vi "Kernel - Command Parser.vi"(7 "data in - Command Parser":T1, 8 "error in":errorcluster, 10 "state":string, 11 "message queue":refnum<queue>) -> (0 "error out":errorcluster, 3 "message queue (out)":refnum<queue>, 4 "stop?":bool, 5 "data out - Command Parser":T1)   [LabVIEW 2021]
uses:
  Typedefs/Data - Command Parser.ctl
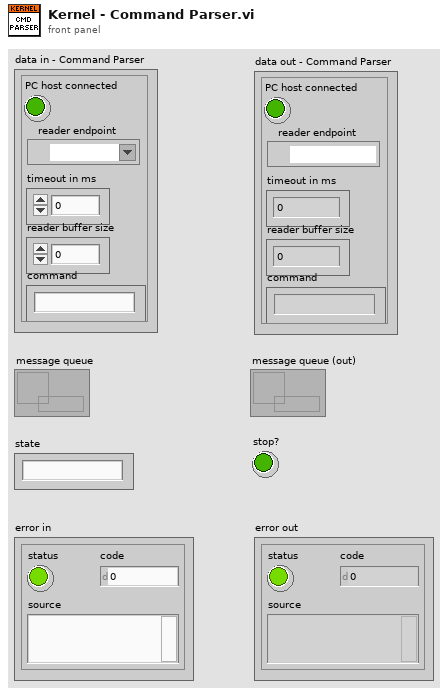
[diagram p1: front panel]
types:
  T1 = typedef "Data - Command Parser.ctl" = cluster{"PC host connected":bool, "timeout in ms":i32, "reader buffer size":i32, "command":string, "reader endpoint":refnum<k21>}
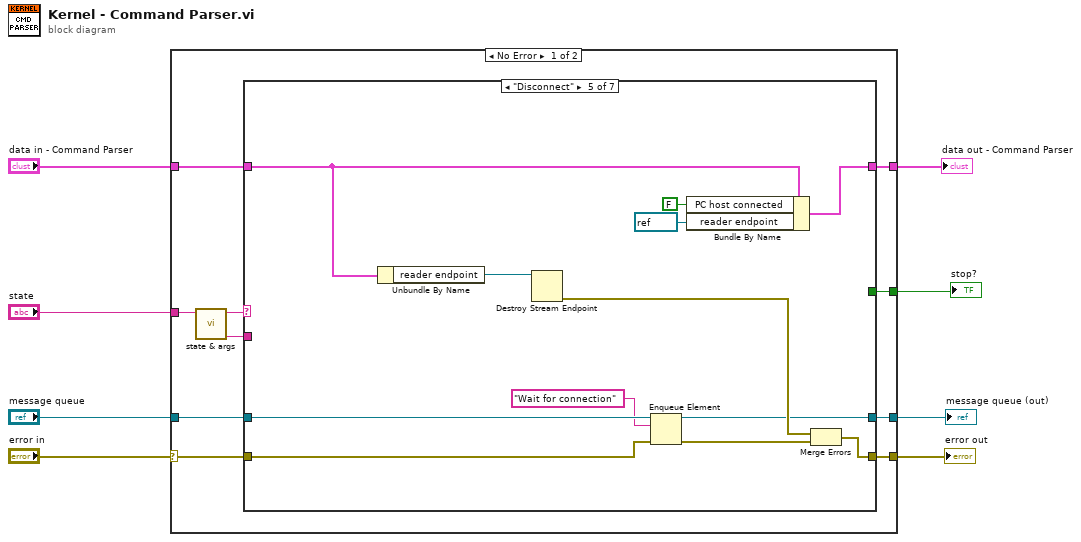
[diagram p0: block diagram]
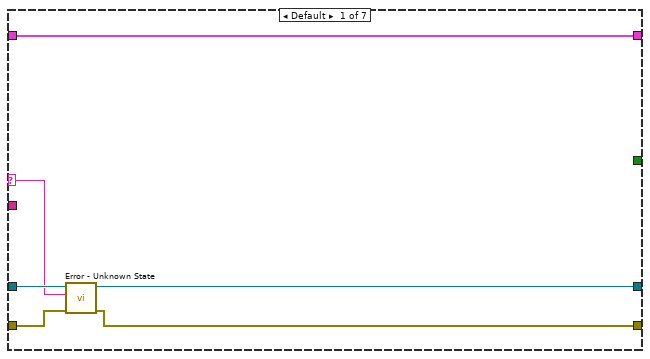
[diagram p2: hidden frame]
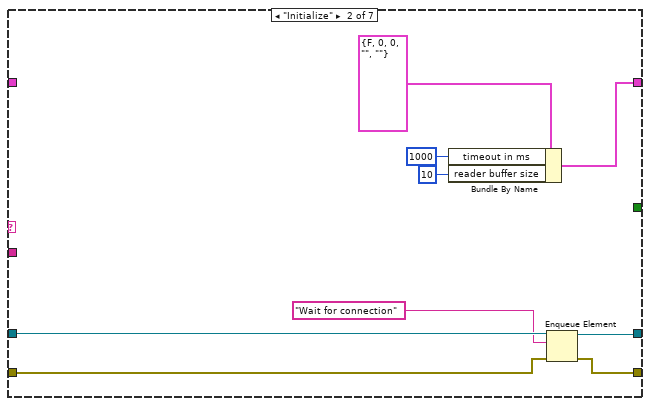
[diagram p3: hidden frame]
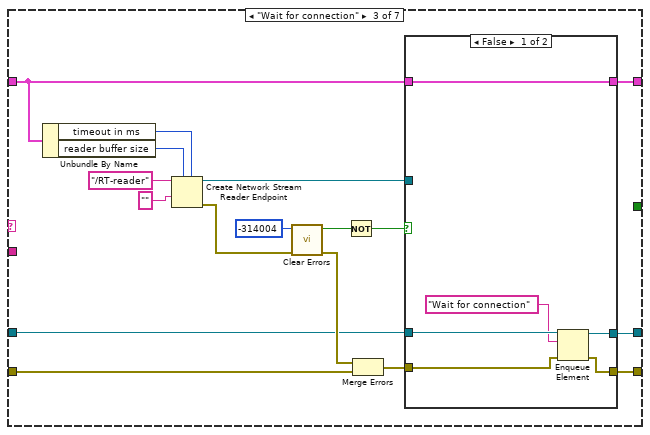
[diagram p4: hidden frame]
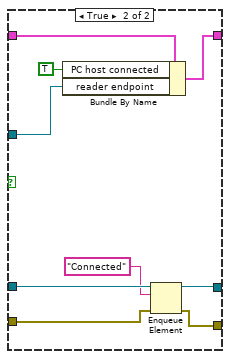
[diagram p5: hidden frame]
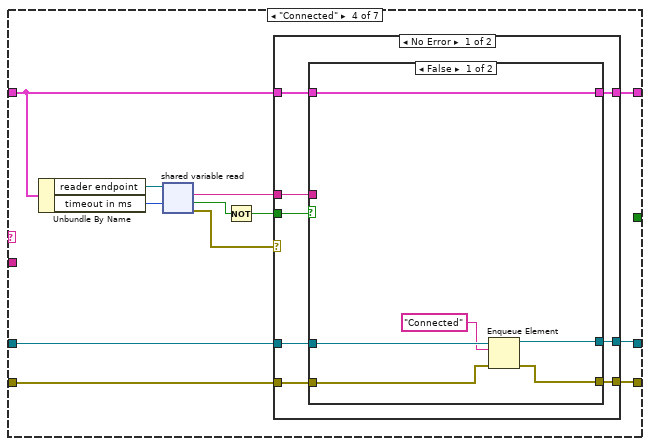
[diagram p6: hidden frame]
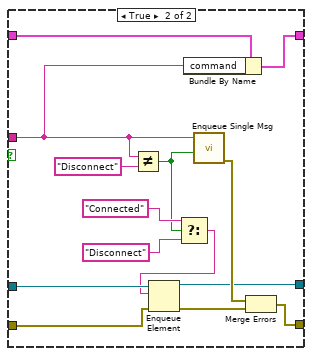
[diagram p7: hidden frame]
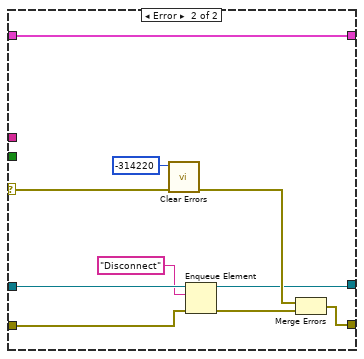
[diagram p8: hidden frame]
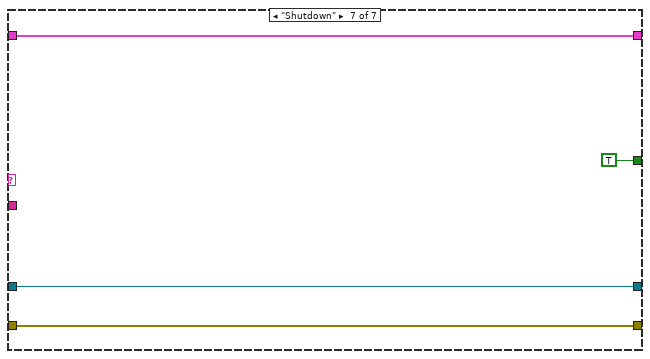
[diagram p10: hidden frame]
diagram:
  n1 = case shown="No Error" "error in" {
    selector: "error in" -> [w17 w135]
    tunnel: "message queue" -> [w18 w136]
    tunnel: "state" -> [w16 _]
    tunnel: "data in - Command Parser" -> [w13 w137]
    tunnel: [w12 w135] -> w4
    tunnel: [w11 w136] -> w3
    tunnel: [w10 w137] -> w2
    tunnel: [w9 _] -> w1
    frame No Error {
      n2 = call "state & args.vi"("state:args"=w16) -> ("args"=w14:string, "state"=w15:string)  [unwired: 9 in]
      n3 = case shown="\"Disconnect\"" w15 {
        selector: w15 -> [w21 _ _ _ _ _ _]
        tunnel: w18 -> [w23 w28 w34 w70 w121 w129 w133]
        tunnel: w17 -> [w24 w27 w39 w69 w117 w128 w134]
        tunnel: w14 -> [_ _ _ _ _ _ _]
        tunnel: w13 -> [w19 _ w49 w77 w124 w130 w132]
        tunnel: [w22 w29 w37 w68 w120 w129 w133] -> w11
        tunnel: [w20 w26 w36 w67 w118 w128 w134] -> w12
        tunnel: [w19 w30 w50 w66 w127 w130 w132] -> w10
        tunnel: [_ _ _ _ _ _ TRUE] -> w9
        frame Default {
          n4 = call "Error - Unknown State.vi"("error in"=w24, "state"=w21, "queue"=w23) -> ("error out"=w20:errorcluster, "queue out"=w22:refnum<queue>)  [unwired: 7 in]
        }
        frame "Initialize" {
          n5 = Bundle By Name(cluster=T1 {"PC host connected"=FALSE, "timeout in ms"=0, "reader buffer size"=0, "command"="", "reader endpoint"=""} ("data in - Command Parser"), "timeout in ms"=1000, "reader buffer size"=10) -> (w30:T1)
          n6 = Enqueue Element(queue=w28, element="Wait for connection", error in (no error)=w27) -> (queue out=w29:refnum<queue>, error out=w26:errorcluster)  [unwired: 1 in, 1 out]
        }
        frame "Wait for connection" {
          n7 = Unbundle By Name(w49) -> ("timeout in ms"=w48:i32, "reader buffer size"=w47:i32)
          n8 = Create Network Stream Reader Endpoint(5:w48, 7:w47, 9:"" ("writer url"), 11:"/RT-reader" ("reader name")) -> (0:w43:errorcluster, 3:w44:refnum<k21>)  [unwired: 3 in]
          n9 = call <vilib>:"Clear Errors.vi"("error in (no error)"=w43, "specific error code to clear (0: all)"=-314004) -> ("error out"=w38:errorcluster, "specific error cleared?"=w41:bool)  [unwired: 4 in]
          n10 = Not(x=w41) -> (.not. x?=w40:bool)
          n11 = Merge Errors(w38, w39) -> (w35:errorcluster)
          n12 = case shown="False" w40 {
            tunnel: w49 -> [w56 w65]
            tunnel: [w56 w64] -> w50
            tunnel: w44 -> [_ w62]
            tunnel: [w55 w61] -> w37
            tunnel: [w54 w58] -> w36
            tunnel: w35 -> [w53 w59]
            tunnel: w34 -> [w52 w60]
            frame False {
              n13 = Enqueue Element(queue=w52, element="Wait for connection", error in (no error)=w53) -> (queue out=w55:refnum<queue>, error out=w54:errorcluster)  [unwired: 1 in, 1 out]
            }
            frame True {
              n14 = Bundle By Name(cluster=w65, "PC host connected"=TRUE, "reader endpoint"=w62) -> (w64:T1)
              n15 = Enqueue Element(queue=w60, element="Connected", error in (no error)=w59) -> (queue out=w61:refnum<queue>, error out=w58:errorcluster)  [unwired: 1 in, 1 out]
            }
          }
        }
        frame "Connected" {
          n16 = Unbundle By Name(w77) -> ("reader endpoint"=w76:refnum<k21>, "timeout in ms"=w75:i32)
          n17 = shared-variable-read(w76, w75) -> (w73:errorcluster, w72:bool, w74:string)  [unwired: 1 in, 1 out]
          n18 = Not(x=w72) -> (.not. x?=w71:bool)
          n19 = case shown="No Error" w73 {
            selector: w73 -> [_ w114]
            tunnel: w77 -> [w82 w115]
            tunnel: w74 -> [w81 _]
            tunnel: w71 -> [w85 _]
            tunnel: w70 -> [w84 w110]
            tunnel: w69 -> [w83 w108]
            tunnel: [w80 w109] -> w68
            tunnel: [w79 w112] -> w67
            tunnel: [w78 w115] -> w66
            frame No Error {
              n20 = case shown="False" w85 {
                tunnel: w84 -> [w90 w104]
                tunnel: w83 -> [w88 w97]
                tunnel: w82 -> [w91 w94]
                tunnel: w81 -> [_ w92]
                tunnel: [w89 w103] -> w80
                tunnel: [w87 w95] -> w79
                tunnel: [w91 w93] -> w78
                frame False {
                  n21 = Enqueue Element(queue=w90, element="Connected", error in (no error)=w88) -> (queue out=w89:refnum<queue>, error out=w87:errorcluster)  [unwired: 1 in, 1 out]
                }
                frame True {
                  n22 = Not Equal?(x=w92, y="Disconnect") -> (x != y?=w99:bool)
                  n23 = Select(t="Connected" ("y"), s=w99, f="Disconnect" ("y")) -> (s? t:f=w98:string)
                  n24 = Enqueue Element(queue=w104, element=w98, error in (no error)=w97) -> (queue out=w103:refnum<queue>, error out=w96:errorcluster)  [unwired: 1 in, 1 out]
                  n25 = Bundle By Name(cluster=w94, "command"=w92) -> (w93:T1)
                  n26 = call "Enqueue Single Msg.vi"("enable (T)"=w99, "queue/message"=w92) -> ("error out"=w105:errorcluster)  [unwired: 9 in]
                  n27 = Merge Errors(w105, w96) -> (w95:errorcluster)
                }
              }
            }
            frame Error {
              n28 = call <vilib>:"Clear Errors.vi"("error in (no error)"=w114, "specific error code to clear (0: all)"=-314220) -> ("error out"=w111:errorcluster)  [unwired: 4 in, 1 out]
              n29 = Enqueue Element(queue=w110, element="Disconnect", error in (no error)=w108) -> (queue out=w109:refnum<queue>, error out=w107:errorcluster)  [unwired: 1 in, 1 out]
              n30 = Merge Errors(w111, w107) -> (w112:errorcluster)
            }
          }
        }
        frame "Disconnect" {
          n31 = Unbundle By Name(w124) -> ("reader endpoint"=w123:refnum<k21>)
          n32 = Destroy Stream Endpoint(11:w123) -> (0:w122:errorcluster)  [unwired: 1 in]
          n33 = Enqueue Element(queue=w121, element="Wait for connection", error in (no error)=w117) -> (queue out=w120:refnum<queue>, error out=w119:errorcluster)  [unwired: 1 in, 1 out]
          n34 = Bundle By Name(cluster=w124, "PC host connected"=FALSE, "reader endpoint"=refnum<k21> refnum) -> (w127:T1)
          n35 = Merge Errors(w122, w119) -> (w118:errorcluster)
        }
        frame "Error" {
        }
        frame "Shutdown" {
        }
      }
    }
    frame Error {
    }
  }
  "error out" <- w4
  "stop?" <- w1
  "message queue (out)" <- w3
  "data out - Command Parser" <- w2
